vi "RT Errors.Set Error Source.vi"(9 "library name (\"\")":string, 10 "vi name":string, 11 "error in":errorcluster) -> (1 "new offset":i32, 3 "error out":errorcluster)   [LabVIEW 2016, in "RT Error Handling.lvlib"]
uses:
  RT Error Handling.lvlib
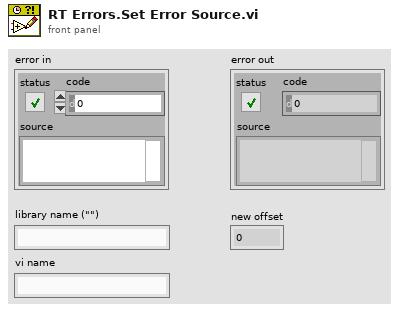
[diagram p1: front panel]
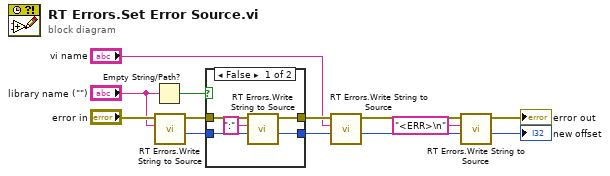
[diagram p0: block diagram]
diagram:
  n1 = Empty String/Path?(string/path="library name (\"\")") -> (empty?=w7:bool)
  n2 = call "RT Errors.Write String to Source.vi"("string"="library name (\"\")", "error in"="error in") -> ("new offset"=w5:i32, "error out"=w6:errorcluster)  [unwired: 8 in]
  n3 = case shown="False" w7 {
    tunnel: w6 -> [w18 w20]
    tunnel: w5 -> [w17 w19]
    tunnel: [w16 w20] -> w4
    tunnel: [w15 w19] -> w3
    frame False {
      n4 = call "RT Errors.Write String to Source.vi"("offset (0)"=w17, "string"=":", "error in"=w18) -> ("new offset"=w15:i32, "error out"=w16:errorcluster)  [unwired: 7 in]
    }
    frame True {
    }
  }
  n5 = call "RT Errors.Write String to Source.vi"("offset (0)"=w3, "string"="vi name", "error in"=w4) -> ("new offset"=w1:i32, "error out"=w9:errorcluster)  [unwired: 7 in]
  n6 = call "RT Errors.Write String to Source.vi"("offset (0)"=w1, "string"="<ERR>\n", "error in"=w9) -> ("new offset"=→"new offset":i32, "error out"=→"error out":errorcluster)  [unwired: 7 in]
